vi "Aircraft Data Router.vi"(7 "Connection Details":T1, 8 "Error In":errorcluster, 10 "Aircraft ID":u8, 11 "MavLINK Message":string) -> (0 "Error Out":errorcluster)   [LabVIEW 2014]
uses:
  Overlord/SubVI/Message Queues/Tx to Overlord/SubVI/Send MAVLink to Overlord.vi
  Controls/Aircraft Discovery State.ctl
  Controls/Known Aircraft.ctl
  SubVI/Queue References/SubVI/Get Aircraft RX Queue String.vi
  SubVI/Queue References/SubVI/Get Aircraft TX Queue String.vi
  Telemetry/Controls/Telemetry Connection Type.ctl
  Hardware Driver/Controls/Coms Driver Interface.ctl
  SubVI/Queue References/SubVI/Get Aircraft Waypoint Queue String.vi
  <vilib>/httpClient/ClientHandle.ctl
  <vilib>/httpClient/LabVIEWHTTPClient.lvlib
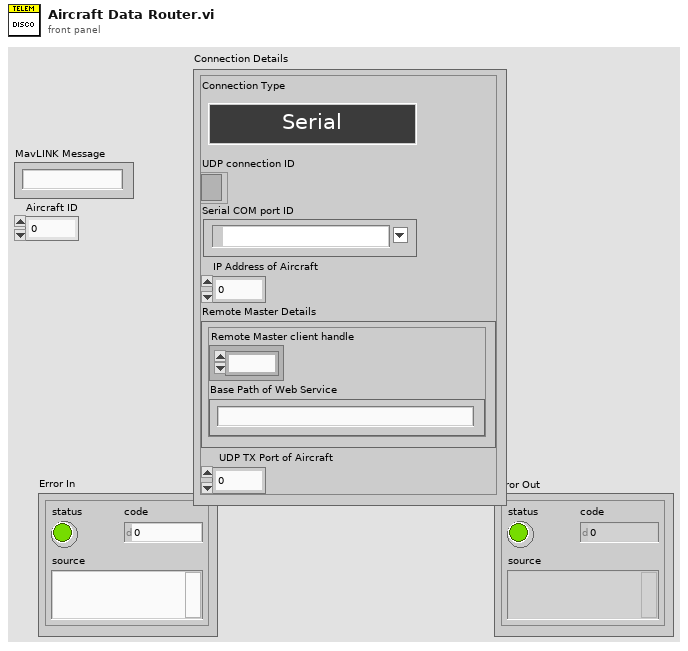
[diagram p1: front panel]
types:
  T1 = typedef "Coms Driver Interface.ctl" = cluster{"Connection Type":T2, "UDP connection ID":refnum<k16>, "Serial COM port ID":refnum<visa-resource-name>, "IP Address of Aircraft":u32, "Remote Master Details":cluster{"Remote Master client handle":T3, "Base Path of Web Service":string}, "UDP TX Port of Aircraft":u16}
  T2 = typedef "Telemetry Connection Type.ctl" = enum16{"Serial", "UDP", "Remote Master"}
  T3 = typedef "LabVIEWHTTPClient.lvlib/ClientHandle.ctl" = refnum<k1>
  T4 = typedef "Aircraft Discovery State.ctl" = enum16{"Initalise", "Check If Known Aircraft", "Route to known coms instance", "Create coms instance for new aircraft", "Complete"}
  T5 = typedef "Known Aircraft.ctl" = cluster{"Aircraft ID":u8, "Aircraft Receive queue Ref":refnum<queue>, "Aircraft Transmit queue Ref":refnum<queue>, "Waypoint Queue Ref":refnum<queue>, "Connection Details":T1}
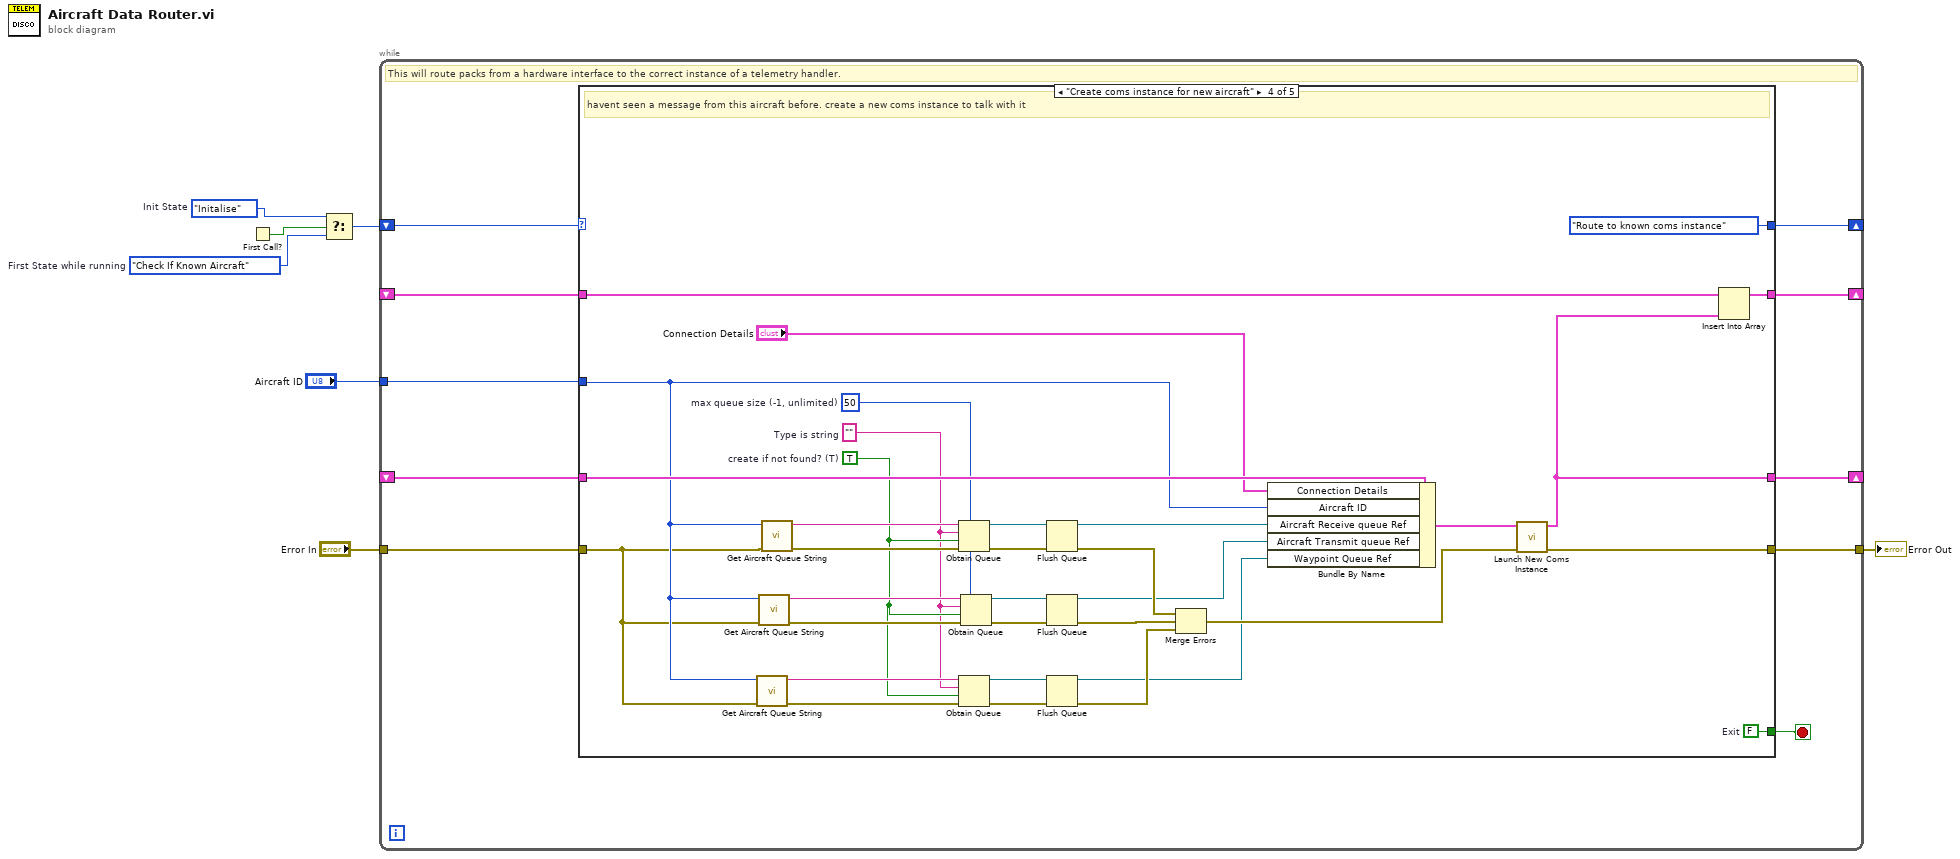
[diagram p0: block diagram]
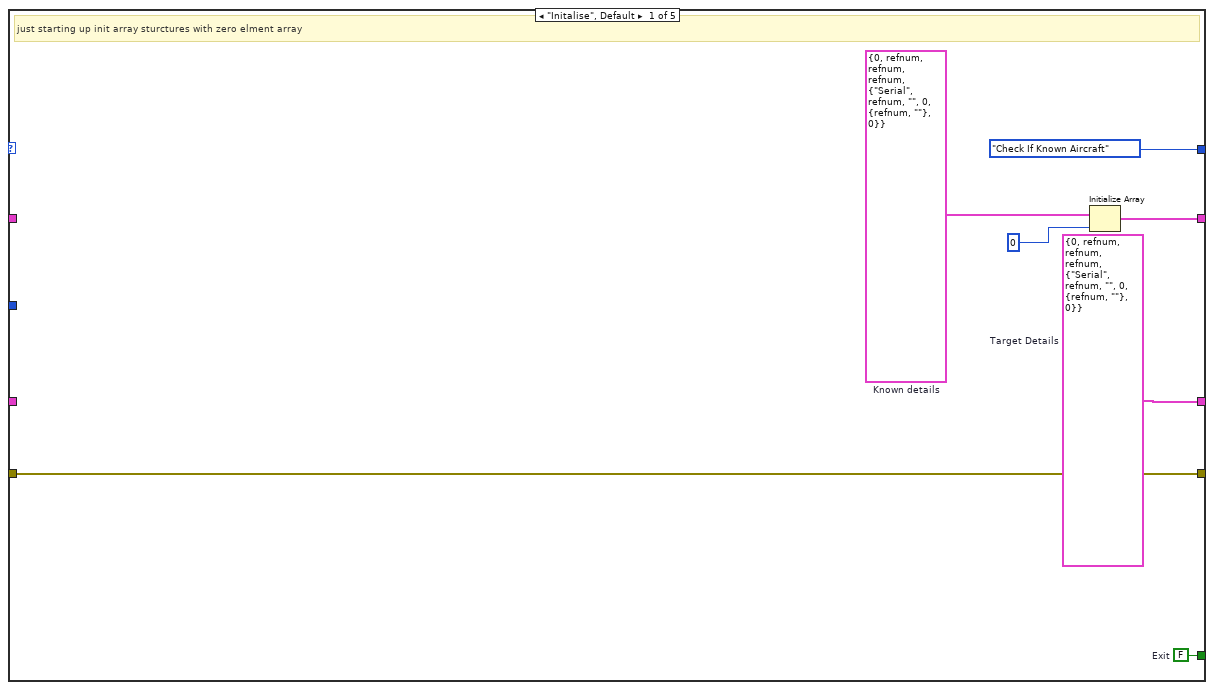
[diagram p2: hidden frame]
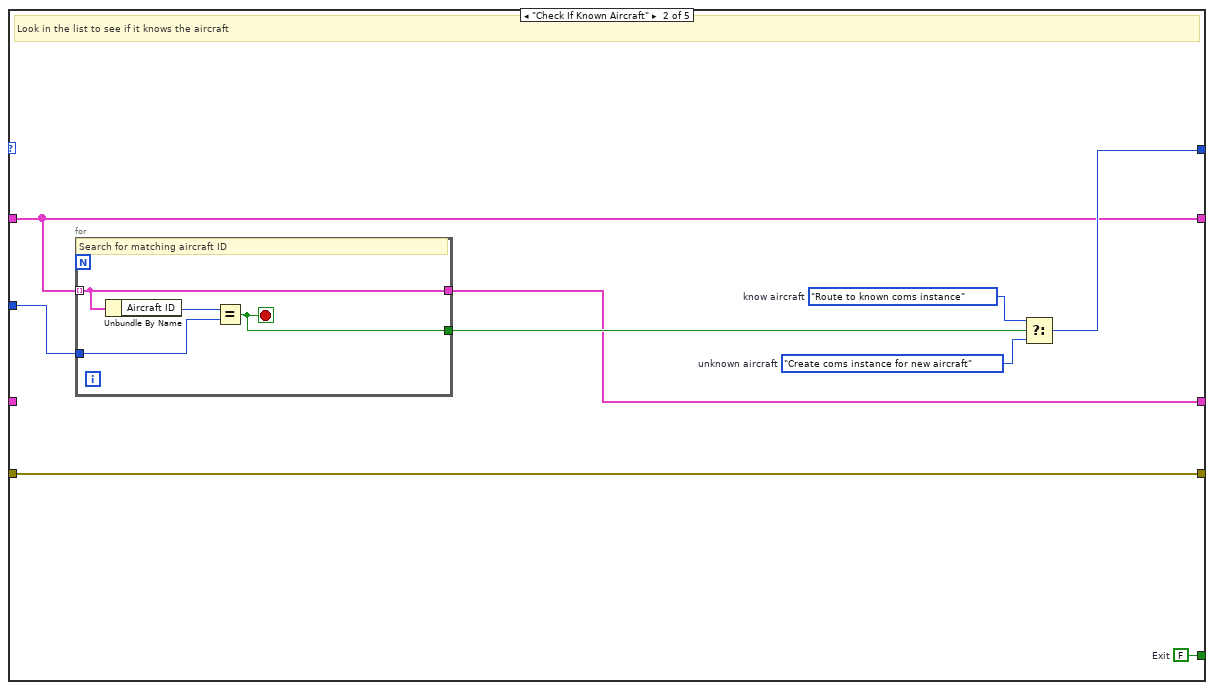
[diagram p3: hidden frame]
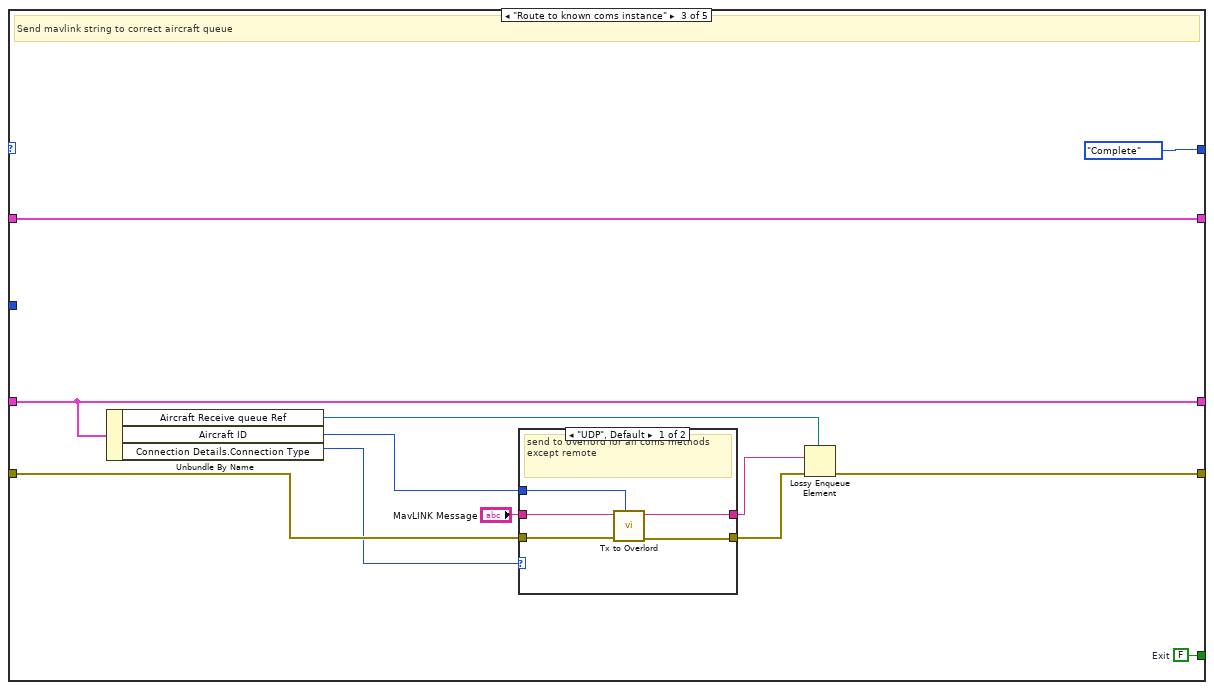
[diagram p4: hidden frame]
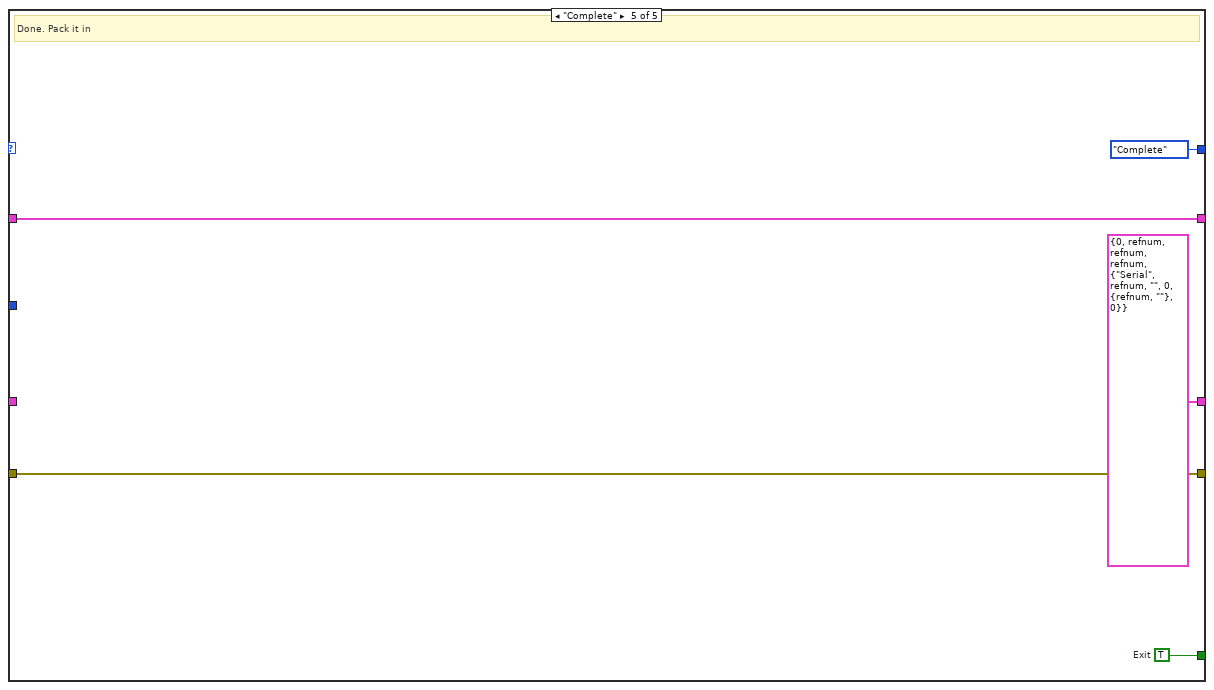
[diagram p6: hidden frame]
diagram:
  w5 = Aircraft_Discovery_State."Check If Known Aircraft"  # First State while running
  w6 = Aircraft_Discovery_State."Initalise"  # Init State
  n1 = First Call?() -> (First Call?: T/F=w1:bool)
  n2 = Select(t=w6, s=w1, f=w5) -> (s? t:f=w4:T4)
  n3 = while {
    tunnel: "Aircraft ID" -> [w17]
    shift-right: [w15] -> _
    shift-left: w4 -> [w16]
    tunnel: "Error In" -> [w14]
    tunnel: [w13] -> w2
    shift-right: [w12] -> _
    shift-left: _ -> [w11]
    shift-right: [w10] -> _
    shift-left: _ -> [w9]
    stop <- w8 stop-if-true
    # "This will route packs from a hardware interface to the correct instance of a telemetry handler."
    n4 = case shown="\"Create coms instance for new aircraft\"" w16 {
      tunnel: w17 -> [_ w28 _ w71 _]
      tunnel: [Aircraft_Discovery_State."Check If Known Aircraft" ("First State while running") w31 Aircraft_Discovery_State."Complete" ("unknown aircraft") Aircraft_Discovery_State."Route to known coms instance" ("unknown aircraft") Aircraft_Discovery_State."Complete" ("unknown aircraft")] -> w15
      tunnel: w14 -> [w23 w30 w44 w67 w88]
      tunnel: [w23 w30 w43 w76 w88] -> w13
      tunnel: [w22 w29 w47 w84 w91] -> w12
      tunnel: w11 -> [_ w29 w47 w85 w91]
      tunnel: [w19 w26 w40 w74 T5 {"Aircraft ID"=0, "Aircraft Receive queue Ref"=refnum, "Aircraft Transmit queue Ref"=refnum, "Waypoint Queue Ref"=refnum, "Connection Details"={"Connection Type"=enum."Serial", "UDP connection ID"=refnum, "Serial COM port ID"="", "IP Address of Aircraft"=0, "Remote Master Details"={"Remote Master client handle"=refnum, "Base Path of Web Service"=""}, "UDP TX Port of Aircraft"=0}} ("Target Details")] -> w10
      tunnel: w9 -> [_ _ w40 w83 _]
      tunnel: [w18 w25 w39 w82 w90] -> w8
      frame "Initalise", Default {
        w18 = FALSE  # Exit
        w19 = T5 {"Aircraft ID"=0, "Aircraft Receive queue Ref"=refnum, "Aircraft Transmit queue Ref"=refnum, "Waypoint Queue Ref"=refnum, "Connection Details"={"Connection Type"=enum."Serial", "UDP connection ID"=refnum, "Serial COM port ID"="", "IP Address of Aircraft"=0, "Remote Master Details"={"Remote Master client handle"=refnum, "Base Path of Web Service"=""}, "UDP TX Port of Aircraft"=0}}  # Target Details
        w21 = T5 {"Aircraft ID"=0, "Aircraft Receive queue Ref"=refnum, "Aircraft Transmit queue Ref"=refnum, "Waypoint Queue Ref"=refnum, "Connection Details"={"Connection Type"=enum."Serial", "UDP connection ID"=refnum, "Serial COM port ID"="", "IP Address of Aircraft"=0, "Remote Master Details"={"Remote Master client handle"=refnum, "Base Path of Web Service"=""}, "UDP TX Port of Aircraft"=0}}  # Known details
        # "just starting up init array sturctures with zero elment array"
        n5 = Initialize Array(w21, 0 ("Known Aircraft ID")) -> (w22:T5[])
      }
      frame "Check If Known Aircraft" {
        w25 = FALSE  # Exit
        w32 = Aircraft_Discovery_State."Create coms instance for new aircraft"  # unknown aircraft
        w33 = Aircraft_Discovery_State."Route to known coms instance"  # know aircraft
        # "Look in the list to see if it knows the aircraft"
        n6 = for {
          tunnel: w29 -> [w34] mode=indexing
          tunnel: w28 -> [w36]
          tunnel: [w35] -> w27
          tunnel: [w34] -> w26
          stop <- w35 stop-if-true
          # "Search for matching aircraft ID"
          n7 = Unbundle By Name(w34) -> ("Aircraft ID"=w37:u8)
          n8 = Equal?(x=w37, y=w36) -> (x = y?=w35:bool)
        }
        n9 = Select(t=w33, s=w27, f=w32) -> (s? t:f=w31:T4)
      }
      frame "Route to known coms instance" {
        w39 = FALSE  # Exit
        # "Send mavlink string to correct aircraft queue"
        n10 = Unbundle By Name(w40) -> ("Aircraft Receive queue Ref"=w42:refnum<queue>, "Aircraft ID"=w45:u8, "Connection Details.Connection Type"=w38:T2)
        n11 = case shown="\"UDP\", Default" w38 {
          tunnel: [w54 w56] -> w49
          tunnel: "MavLINK Message" -> [w53 w55]
          tunnel: w45 -> [w52 _]
          tunnel: w44 -> [w51 w56]
          tunnel: [w50 w55] -> w41
          frame "UDP", Default {
            # "send to overlord for all coms methods except remote"
            n12 = call-poly "Tx to Overlord.vi"("Aircraft ID"=w52, "Error In"=w51, "MAVLink String"=w53) -> ("error out"=w54:errorcluster, "MAVLink String Out"=w50:string)  [unwired: 7 in]
          }
          frame "Remote Master" {
            # "Dont send to overlord if in remote master mode (would just be feedback)"
          }
        }
        n13 = Lossy Enqueue Element(queue=w42, element=w41, error in (no error)=w49) -> (error out=w43:errorcluster)  [unwired: 3 out]
      }
      frame "Create coms instance for new aircraft" {
        w82 = FALSE  # Exit
        w66 = TRUE  # create if not found? (T)
        w80 = 50  # max queue size (-1, unlimited)
        w65 = ""  # Type is string
        # "havent seen a message from this aircraft before. create a new coms instance to talk with it"
        n14 = call-poly "Get Aircraft Queue String.vi"("Error In"=w67, "Aircraft ID"=w71) -> ("Error Out"=w68:errorcluster, "Aircraft Queue Name"=w72:string)  [unwired: 8 in]
        n15 = call-poly "Get Aircraft Queue String.vi"("Error In"=w67, "Aircraft ID"=w71) -> ("Error Out"=w69:errorcluster, "Aircraft Queue Name"=w81:string)  [unwired: 8 in]
        n16 = call-poly "Get Aircraft Queue String.vi"("Error In"=w67, "Aircraft ID"=w71) -> ("Error Out"=w70:errorcluster, "Aircraft Q Name"=w86:string)  [unwired: 8 in]
        n17 = Obtain Queue(max queue size (-1, unlimited)=w80, name (unnamed)=w86, element data type=w65, create if not found? (T)=w66, error in (no error)=w70) -> (queue out=w62:refnum<queue>, error out=w60:errorcluster)  [unwired: 1 out]
        n18 = Obtain Queue(name (unnamed)=w72, element data type=w65, create if not found? (T)=w66, error in (no error)=w68) -> (queue out=w63:refnum<queue>, error out=w64:errorcluster)  [unwired: 1 in, 1 out]
        n19 = Obtain Queue(max queue size (-1, unlimited)=w80, name (unnamed)=w81, element data type=w65, create if not found? (T)=w66, error in (no error)=w69) -> (queue out=w78:refnum<queue>, error out=w79:errorcluster)  [unwired: 1 out]
        n20 = Flush Queue(queue=w62, error in (no error)=w60) -> (queue out=w61:refnum<queue>, error out=w59:errorcluster)  [unwired: 1 out]
        n21 = Flush Queue(queue=w78) -> (queue out=w58:refnum<queue>)  [unwired: 1 in, 2 out]
        n22 = Flush Queue(queue=w63) -> (queue out=w57:refnum<queue>)  [unwired: 1 in, 2 out]
        n23 = Merge Errors(w59, w79, w64) -> (w77:errorcluster)
        n24 = Bundle By Name(cluster=w83, "Connection Details"="Connection Details", "Aircraft ID"=w71, "Aircraft Receive queue Ref"=w61, "Aircraft Transmit queue Ref"=w58, "Waypoint Queue Ref"=w57) -> (w75:T5)
        n25 = call "Launch New Coms Instance.vi"("Error In"=w77, "Instance Details"=w75) -> ("Error Out"=w76:errorcluster, "Instance Details Out"=w74:T5)  [unwired: 8 in]
        n26 = Insert Into Array(array=w85, new element=w74) -> (w84:T5[])  [unwired: 1 in]
      }
      frame "Complete" {
        w90 = TRUE  # Exit
        # "Done. Pack it in"
      }
    }
  }
  "Error Out" <- w2
